vi "AutoAlign_SWITCH.vi"() -> ()   [LabVIEW 2014]
doc: "This example shows how to make a simple VI that views VIs. Although it runs and aborts the VIs that it displays, this\nis not necessary. Any VIs that are aborted will need to be designed with this in mind. For VIs that cannot be aborted, please see the communication example."
panel:
  in  "Select a VI":T1(radio)
  in  "Stop":bool
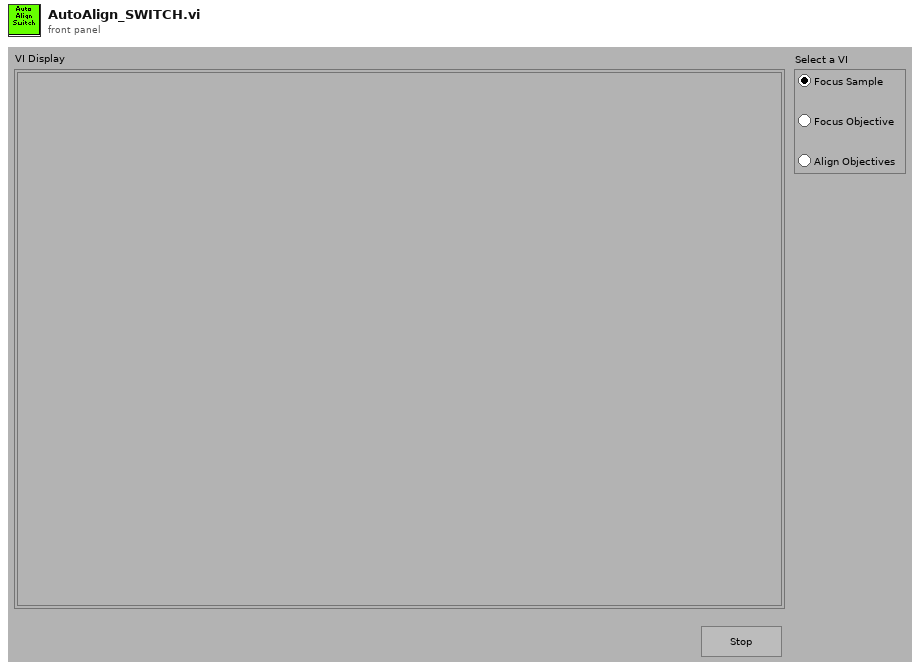
[diagram p1: front panel]
types:
  T1 = enum32{"DC Mike Control", "Radio Selection 2", "Radio Selection 3"}
  T2 = enum32{"Bad", "Idle", "Run top level", "Running"}
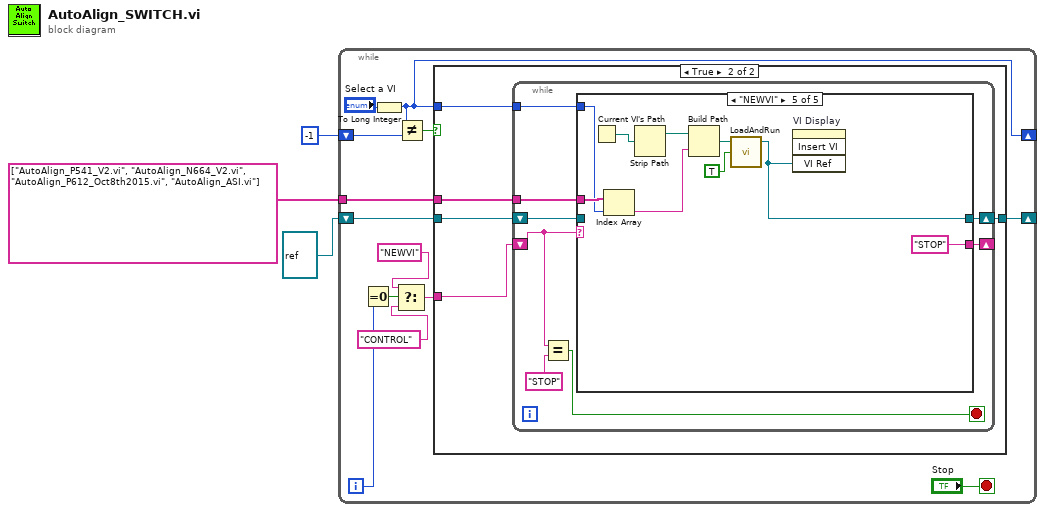
[diagram p0: block diagram]
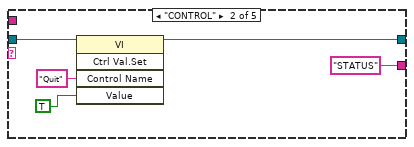
[diagram p4: hidden frame]
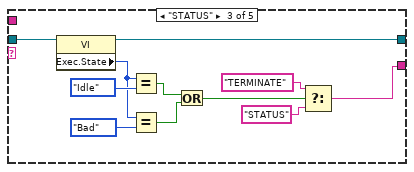
[diagram p5: hidden frame]
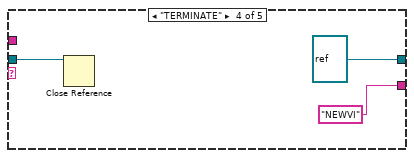
[diagram p6: hidden frame]
diagram:
  n1 = while {
    tunnel: string[] ["AutoAlign_P541_V2.vi", "AutoAlign_N664_V2.vi", "AutoAlign_P612_Oct8th2015.vi", "AutoAlign_ASI.vi"] -> [w15]
    shift-right: [w10] -> _
    shift-left: refnum<vi> refnum ("VI Ref") -> [w14]
    shift-right: [w9] -> _
    shift-left: -1 -> [w12]
    i -> [w8]
    stop <- "Stop" stop-if-true
    n2 = Equal To 0?(x=w8) -> (x = 0?=w7:bool)
    n3 = To Long Integer(number="Select a VI") -> (32bit integer=w9:i32)
    n4 = Select(t="NEWVI" ("Control Name"), s=w7, f="CONTROL" ("Control Name")) -> (s? t:f=w4:string)
    n5 = Not Equal?(x=w9, y=w12) -> (x != y?=w13:bool)
    n6 = case shown="True" w13 {
      tunnel: w15 -> [_ w22]
      tunnel: w14 -> [w17 w21]
      tunnel: [w17 w20] -> w10
      tunnel: w9 -> [_ w19]
      tunnel: w4 -> [_ w18]
      frame False {
      }
      frame True {
        n7 = while {
          tunnel: w22 -> [w30]
          tunnel: w19 -> [w27]
          shift-right: [w23] -> _
          shift-left: w18 -> [w25]
          shift-right: [w28] -> w20
          shift-left: w21 -> [w29]
          stop <- w24 stop-if-true
          n8 = Equal?(x=w25, y="STOP" ("Control Name")) -> (x = y?=w24:bool)
          n9 = case shown="\"NEWVI\"" w25 {
            selector: w25 -> [w31 _ _ _ _]
            tunnel: w30 -> [_ _ _ _ w60]
            tunnel: w29 -> [w32 w37 w48 w51 _]
            tunnel: [w32 w34 w47 refnum<vi> refnum ("VI Ref") w52] -> w28
            tunnel: w27 -> [_ _ _ _ w55]
            tunnel: [w31 "STATUS" w44 "NEWVI" ("Control Name") "STOP" ("Control Name")] -> w23
            frame "STOP", Default {
            }
            frame "CONTROL" {
              n10 = invoke class="VI" method="Ctrl Val.Set"(reference=w37, "Control Name"="Quit", "Value"=TRUE) -> (reference out=w34:refnum<vi>)  [unwired: 2 in, 4 out]
            }
            frame "STATUS" {
              n11 = property class="VI"(reference=w48) -> (reference out=w47:refnum<vi>, "Exec.State"=w41:T2)  [unwired: 1 in, 1 out]
              n12 = Equal?(x=w41, y=T2."Idle") -> (x = y?=w39:bool)
              n13 = Equal?(x=w41, y=T2."Bad") -> (x = y?=w38:bool)
              n14 = Or(x=w39, y=w38) -> (x .or. y?=w40:bool)
              n15 = Select(t="TERMINATE" ("Control Name"), s=w40, f="STATUS" ("Control Name")) -> (s? t:f=w44:string)
            }
            frame "TERMINATE" {
              n16 = Close Reference(reference=w51) -> ()  [unwired: 1 in, 1 out]
            }
            frame "NEWVI" {
              n17 = Current VI's Path() -> (path=w59:path)
              n18 = Index Array(array=w60, index=w55) -> (element=w53:string)
              n19 = Strip Path(path=w59) -> (stripped path=w58:path)  [unwired: 1 out]
              n20 = Build Path(base path=w58, name or relative path=w53) -> (appended path=w57:path)
              n21 = call "LoadAndRun.vi"("run?"=TRUE, "path"=w57) -> ("vi refnum out"=w52:refnum<vi>)  [unwired: 2 in, 1 out]
              n22 = invoke on="VI Display" class="SubPanel" method="Insert VI"("VI Ref"=w52) -> ()  [unwired: 3 in, 4 out]
            }
          }
        }
      }
    }
  }
